vi "6-18.vi"() -> ()   [LabVIEW 2017]
panel:
  out "Waveform Chart":dynamicdata(graph)
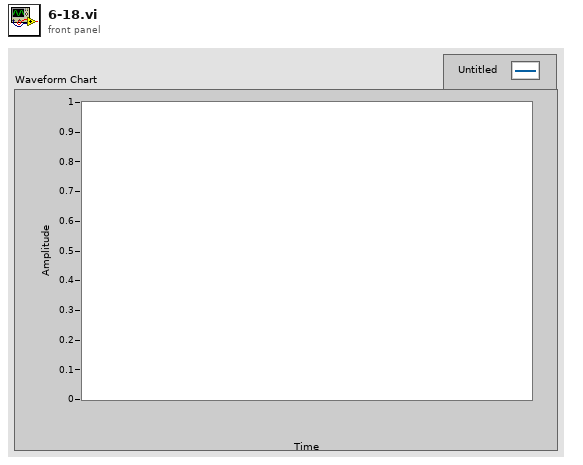
[diagram p1: front panel]
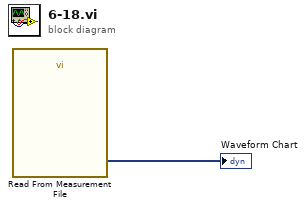
[diagram p0: block diagram]
diagram:
  n1 = call "Read From Measurement File"() -> ("Signals"=→"Waveform Chart":dynamicdata)  [unwired: 6 in, 5 out]
